vi "Dequeue Published Result by Method.vi"(8 "error in (no error)":errorcluster, 9 "timeout in ms":i32, 10 "Method Name":string, 11 "Mock Result Observer In":refnum<class "Mock Result Observer.lvclass">) -> (0 "error out":errorcluster, 1 "timed out?":bool, 2 "Result":T1={"Name"="", "Message"="", "Description"="", "Status"=enum."Passed", "Result Type"=enum."Test Case", "Execution Time"=0.0}, 3 "Mock Result Observer Out":refnum<class "Mock Result Observer.lvclass">)   [LabVIEW 2020, in "Mock Result Observer.lvclass"]
uses:
  Mock Result Observer.lvclass
  source/Core/Result/Result.ctl
  source/Core/Result/Status.ctl
  source/Core/Result/Type.ctl
  source/Core/Result/Result.lvlib
panel:
  out "Array":string[](array[string])
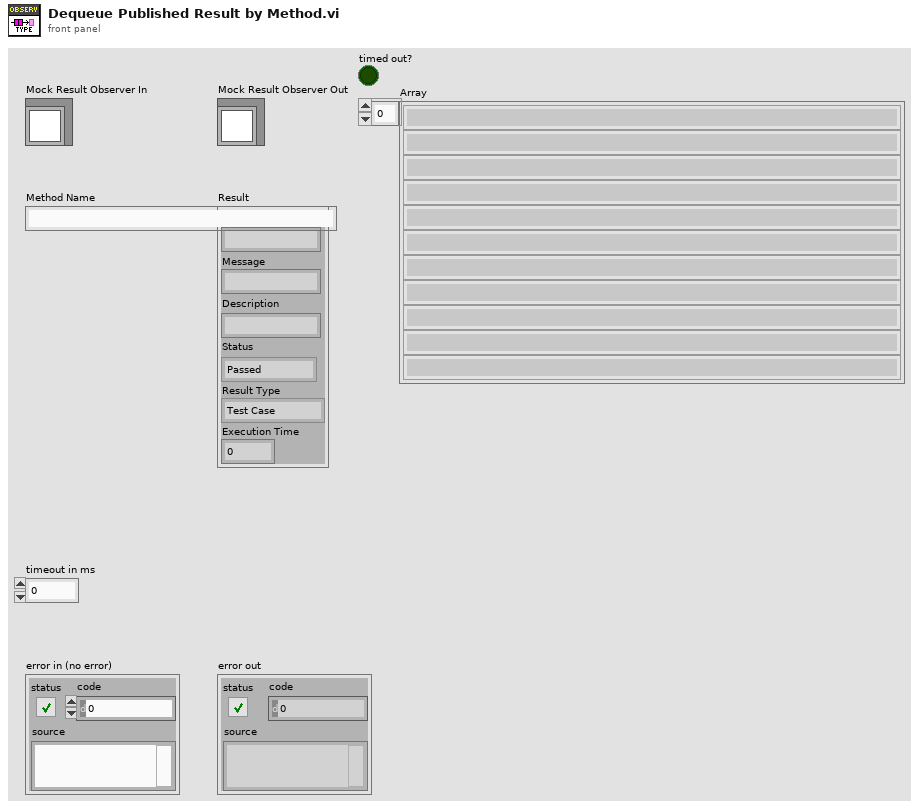
[diagram p1: front panel]
types:
  T1 = typedef "Result.lvlib/Result.ctl" = cluster{"Name":string, "Message":string, "Description":string, "Status":T2, "Result Type":T3, "Execution Time":dbl}
  T2 = typedef "Result.lvlib/Status.ctl" = enum16{"", "Passed", "Failed", "Error", "Skipped", "Setup Error", "Broken", "Teardown Error"}
  T3 = typedef "Result.lvlib/Type.ctl" = enum16{"Test Case", "Test Suite", "Test Run", "Pass", "Fail", "Skip", "Pass if", "Fail if", "Pass if Error", "Fail if Error", "Pass if Equal", "Fail if Equal"}
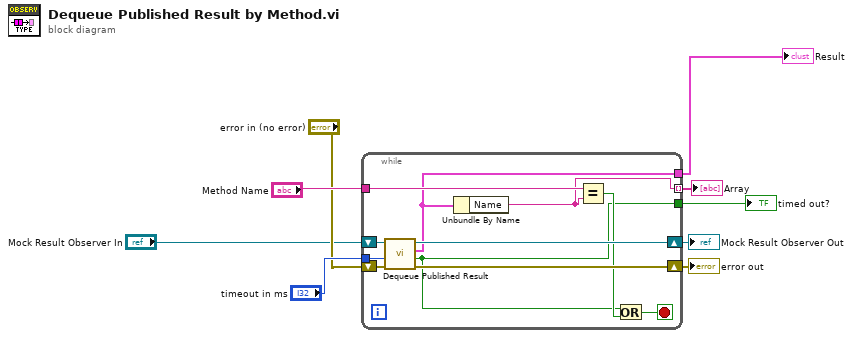
[diagram p0: block diagram]
diagram:
  n1 = while {
    tunnel: "timeout in ms" -> [w16]
    shift-right: [w20] -> w3
    shift-left: "Mock Result Observer In" -> [w18]
    shift-right: [w19] -> w4
    shift-left: "error in (no error)" -> [w17]
    tunnel: "Method Name" -> [w15]
    tunnel: [w12] -> w9
    tunnel: [w11] -> w2
    tunnel: [w10] -> w1 mode=indexing
    stop <- w14 stop-if-true
    n2 = call "Dequeue Published Result.vi"("error in (no error)"=w17, "timeout in ms (-1)"=w16, "Mock Result Observer In"=w18) -> ("error out"=w19:errorcluster, "timed out?"=w11:bool, "Result"=w12:T1, "Mock Result Observer Out"=w20:refnum<class "Mock Result Observer.lvclass">)  [unwired: 5 in]
    n3 = Unbundle By Name(w12) -> ("Name"=w10:string)
    n4 = Equal?(x=w15, y=w10) -> (x = y?=w13:bool)
    n5 = Or(x=w11, y=w13) -> (x .or. y?=w14:bool)
  }
  "Result" <- w9
  "error out" <- w4
  "Mock Result Observer Out" <- w3
  "timed out?" <- w2
  "Array" <- w1
